vi "RegressionDifferentiator.vi"(8 "y":dbl[](array[numeric]), 9 "x":dbl[](array[numeric]), 11 "Interpolation Order":dbl=nan) -> (0 "P''(x)":dbl[](array[numeric]) min=0.0 max=127.0 format="%#.6g", 1 "P(x)":T2, 2 "Integral P(x)":dbl[](array[numeric]) min=0.0 max=127.0 format="%#.6g", 3 "Mode":T1(ring), 4 "integral of P(x)":dbl, 6 "P'(x)":dbl[](array[numeric]) min=0.0 max=127.0 format="%#.6g")   [LabVIEW 2025]
doc: "Computes coefficients for a polynomial (and its derivative) that fits a least squares regression or a perfect interpolation to the provided data. If the Regression Order is unwired, the polynomial of the lowest order that perfectly interpolates the data will be used. \n\nA Mode flag is available so that the user can know if a regression or interpolation was used.\n\nIf the user tries to fit a too-high order polynomial to the data, the method will fail without error, and the Mode flag will reflect this.\n\nAlso outputs the integral of P(x) over [a,b] where a and b are the first and last elements in the x array"
uses:
  <vilib>/Analysis/Matrix/Datatypes/RealMatrix.ctl
  <vilib>/Analysis/baseanly.llb/Real A x B.vi
  <vilib>/Analysis/Matrix/Numeric/Conversions/Array To Matrix - RA2.vi
  <vilib>/Analysis/7linalg.llb/Create Special Real Matrix.vi
  <vilib>/Analysis/7linalg.llb/Solve Linear Equations (multiple right hand).vi
  <vilib>/Analysis/Matrix/Numeric/Conversions/Array To Matrix - RA.vi
  <vilib>/Analysis/Matrix/Numeric/Conversions/Matrix To Array - RM.vi
  <vilib>/Analysis/polynomials.llb/Indefinite Integral of Polynomial (DBL).vi
  <vilib>/Analysis/polynomials.llb/Polynomial Plot (Range).vi
  <vilib>/Analysis/polynomials.llb/nth Derivative of Polynomial (DBL).vi
  <vilib>/Analysis/NI_AALPro.lvlib
  <vilib>/Analysis/Matrix/NI_Matrix.lvlib
  <vilib>/Analysis/NI_AALBase.lvlib
panel:
  out "?":cluster{"X":dbl[], "Real 2D Array":dbl[]}[](graph)
  out "X (Vandermone Matrix)":T2
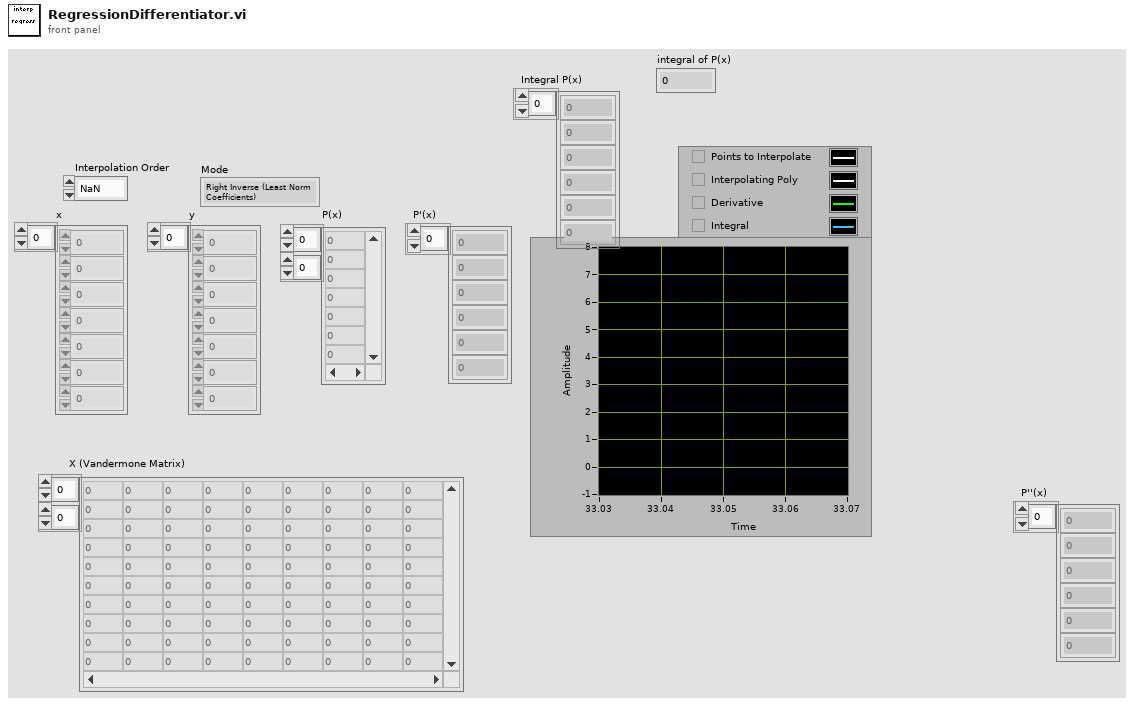
[diagram p1: front panel]
types:
  T1 = enum16{"Right Inverse (Least Norm Coefficients)", "Interpolation", "Regression"}
  T2 = typedef "NI_Matrix.lvlib/RealMatrix.ctl" = dbl[][]
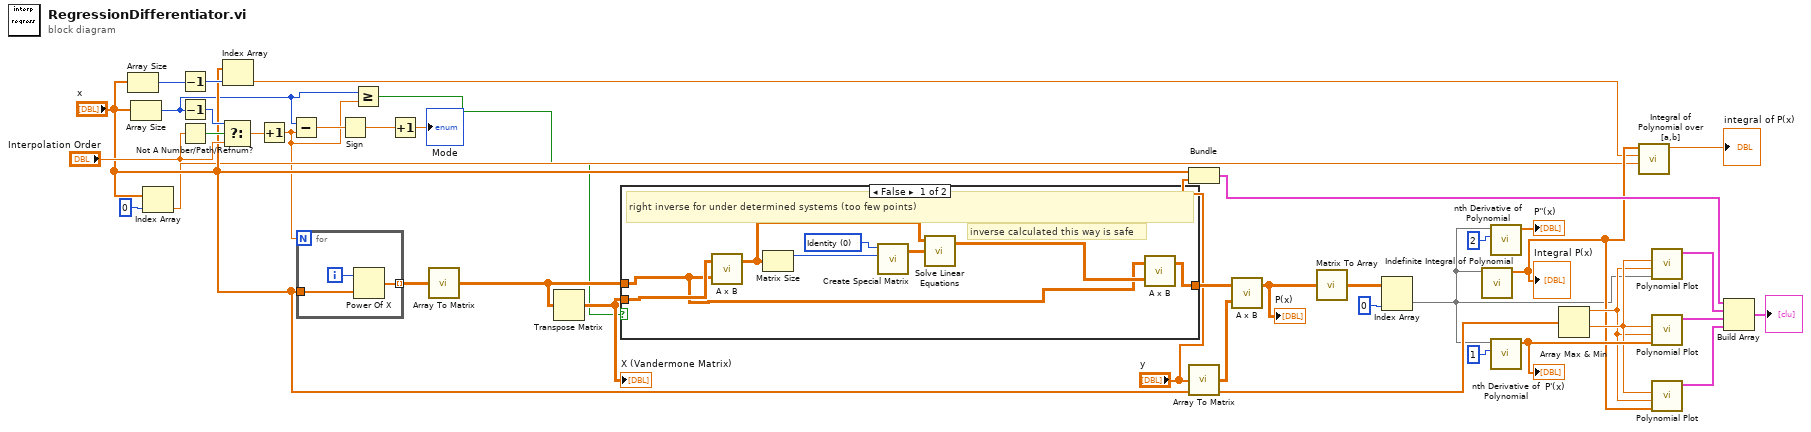
[diagram p0: block diagram]
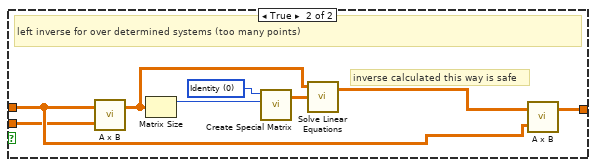
[diagram p2: hidden frame]
diagram:
  n1 = Array Size(array="x") -> (size(s)=w15:i32)
  n2 = Array Size(array="x") -> (size(s)=w3:i32)
  n3 = Index Array(array="x", index=0) -> (element=w8:dbl)
  n4 = Decrement(x=w15) -> (x-1=w14:i32)
  n5 = Decrement(x=w3) -> (x-1=w19:i32)
  n6 = Not A Number/Path/Refnum?(number/path/refnum="Interpolation Order") -> (NaN/Path/Refnum?=w22:bool)
  n7 = Select(t=w19, s=w22, f="Interpolation Order") -> (s? t:f=w20:dbl)
  n8 = Index Array(array="x", index=w14) -> (element=w9:dbl)
  n9 = Increment(x=w20) -> (x+1=w2:dbl)
  n10 = Subtract(x=w3, y=w2) -> (x-y=w25:dbl)
  n11 = for {
    N: w2 -> [_]
    tunnel: "x" -> [w42]
    tunnel: [w40] -> w39 mode=indexing
    i -> [w41]
    n12 = Power Of X(1:w42, 2:w41) -> (0:w40:dbl[])
  }
  n13 = Sign(1:w25) -> (0:w24:dbl)
  n14 = Greater Or Equal?(x=w3, y=w2) -> (x >= y?=w1:bool)
  n15 = Increment(x=w24) -> (x+1=→"Mode":dbl)
  n16 = call-poly <vilib>:"Array To Matrix.vi"("Real 2D Array"=w39) -> ("Real Matrix"=w38:T2)
  n17 = Transpose Matrix(1:w38) -> (0:w7:T2)
  "X (Vandermone Matrix)" <- w7
  n18 = case shown="False" w1 {
    tunnel: w38 -> [w43 w58]
    tunnel: [w44 w57] -> w37
    tunnel: w7 -> [w46 w53]
    frame False {
      w47 = 0 items=["Identity", "Diagonal", "Toeplitz", "Vandermonde", "Companion", "Hankel", "Hadamard", "Wilkinson", "Hilbert", "Inverse Hilbert", "Rosser", "Pascal"] ("matrix type")
      # "inverse calculated this way is safe"
      # "right inverse for under determined systems (too few points)"
      n19 = call-poly <vilib>:"A x B.vi"("B"=w43, "A"=w46) -> ("A x B"=w50:T2)  [unwired: 1 out]
      n20 = Matrix Size(0:w50) -> (1:w48:i32)  [unwired: 1 out]
      n21 = call-poly <vilib>:"Create Special Matrix.vi"("matrix type"=w47, "matrix size"=w48) -> ("Special Matrix"=w49:T2)  [unwired: 3 in, 1 out]
      n22 = call-poly <vilib>:"Solve Linear Equations.vi"("Known Matrix"=w49, "Input Matrix"=w50) -> ("Solution Matrix"=w45:T2)  [unwired: 1 in, 1 out]
      n23 = call-poly <vilib>:"A x B.vi"("B"=w45, "A"=w43) -> ("A x B"=w44:T2)  [unwired: 1 out]
    }
    frame True {
      w56 = 0 items=["Identity", "Diagonal", "Toeplitz", "Vandermonde", "Companion", "Hankel", "Hadamard", "Wilkinson", "Hilbert", "Inverse Hilbert", "Rosser", "Pascal"] ("matrix type")
      # "inverse calculated this way is safe"
      # "left inverse for over determined systems (too many points)"
      n24 = call-poly <vilib>:"A x B.vi"("B"=w53, "A"=w58) -> ("A x B"=w51:T2)  [unwired: 1 out]
      n25 = Matrix Size(0:w51) -> (1:w55:i32)  [unwired: 1 out]
      n26 = call-poly <vilib>:"Create Special Matrix.vi"("matrix type"=w56, "matrix size"=w55) -> ("Special Matrix"=w54:T2)  [unwired: 3 in, 1 out]
      n27 = call-poly <vilib>:"Solve Linear Equations.vi"("Known Matrix"=w54, "Input Matrix"=w51) -> ("Solution Matrix"=w52:T2)  [unwired: 1 in, 1 out]
      n28 = call-poly <vilib>:"A x B.vi"("B"=w58, "A"=w52) -> ("A x B"=w57:T2)  [unwired: 1 out]
    }
  }
  n29 = Bundle("x"="x", "y"="y") -> (w35:cluster{"x":dbl[], "y":dbl[]})  [unwired: 1 in]
  n30 = call-poly <vilib>:"Array To Matrix.vi"("Real 1D Array"="y") -> ("Real Matrix (Column Vector)"=w36:T2)
  n31 = call-poly <vilib>:"A x B.vi"("B"=w36, "A"=w37) -> ("A x B"=w27:T2)  [unwired: 1 out]
  "P(x)" <- w27
  n32 = call-poly <vilib>:"Matrix To Array.vi"("Real Matrix"=w27) -> ("Real 2D Array"=w32:dbl[][])
  n33 = Index Array(array=w32, index (col)=0 ("disabled index (col)")) -> (element=w4:dbl[])  [unwired: 1 in]
  n34 = call-poly <vilib>:"Indefinite Integral of Polynomial.vi"("P(x)"=w4) -> ("Indefinite Integral of P(x)"=w11:dbl[])  [unwired: 9 in, 1 out]
  "Integral P(x)" <- w11
  n35 = call-poly <vilib>:"nth Derivative of Polynomial.vi"("order"=2, "P(x)"=w4) -> ("Nth Derivative of P(x)"=→"P''(x)":dbl[])  [unwired: 8 in, 1 out]
  n36 = call-poly <vilib>:"nth Derivative of Polynomial.vi"("order"=1, "P(x)"=w4) -> ("Nth Derivative of P(x)"=w28:dbl[])  [unwired: 8 in, 1 out]
  "P'(x)" <- w28
  n37 = Array Max & Min(array="x") -> (max value=w17:dbl, min value=w18:dbl)  [unwired: 2 out]
  n38 = call <vilib>:"Integral of Polynomial over [a,b].vi"("b"=w8, "a"=w9, "P(x)"=w11) -> ("integral of P(x)"=→"integral of P(x)":dbl)  [unwired: 7 in, 1 out]
  n39 = call-poly <vilib>:"Polynomial Plot.vi"("P(x)"=w4, "end"=w17, "start"=w18) -> ("polynomial plot"=w26:cluster{"Ramp Pattern":dbl[], "P(A)":dbl[]})  [unwired: 7 in, 1 out]
  n40 = call-poly <vilib>:"Polynomial Plot.vi"("P(x)"=w28, "end"=w17, "start"=w18) -> ("polynomial plot"=w29:cluster{"Ramp Pattern":dbl[], "P(A)":dbl[]})  [unwired: 7 in, 1 out]
  n41 = call-poly <vilib>:"Polynomial Plot.vi"("P(x)"=w11, "end"=w17, "start"=w18) -> ("polynomial plot"=w16:cluster{"Ramp Pattern":dbl[], "P(A)":dbl[]})  [unwired: 7 in, 1 out]
  n42 = Build Array(w35, w26, w29, w16) -> (→"?":cluster{"Ramp Pattern":dbl[], "P(A)":dbl[]}[])
